vi "ex8.vi"() -> ()   [LabVIEW 2022 SP3]
panel:
  out "Out":string
  in  "IN":string
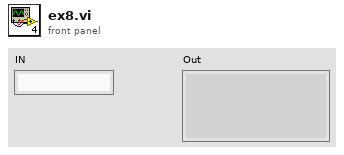
[diagram p1: front panel]
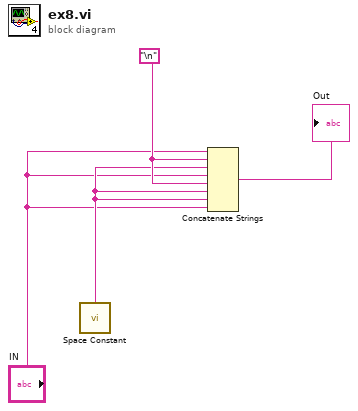
[diagram p0: block diagram]
diagram:
  w3 = "\n"
  n1 = call <vilib>:"Space Constant.vi"() -> ("String"=w2:string)
  n2 = Concatenate Strings("IN", w3, w2, "IN", w3, w2, w2, "IN") -> (→"Out":string)
